vi "RichToFlatni_measurementlink_pinmap_v1_PinGroupDefinition.vi"(5 "OutputClusterType":T1, 11 "InputCluster":T2) -> (3 "OutputCluster":T1)   [LabVIEW 2021, in "ni.measurementlink.pinmap.v1.api.lvlib"]
uses:
  ni.measurementlink.pinmap.v1.api.lvlib
  ni_measurementlink_pinmap_v1_PinGroupDefinition.ctl
  ni_measurementlink_pinmap_v1_PinGroupDefinition_Flat.ctl
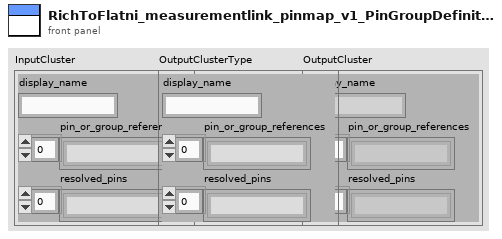
[diagram p1: front panel]
types:
  T1 = typedef "ni.measurementlink.pinmap.v1.api.lvlib/ni_measurementlink_pinmap_v1_PinGroupDefinition_Flat.ctl" = cluster{"display_name":string, "pin_or_group_references":string[], "resolved_pins":string[]}
  T2 = typedef "ni.measurementlink.pinmap.v1.api.lvlib/ni_measurementlink_pinmap_v1_PinGroupDefinition.ctl" = cluster{"display_name":string, "pin_or_group_references":string[], "resolved_pins":string[]}
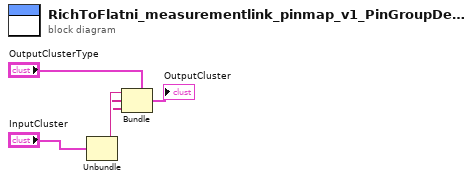
[diagram p0: block diagram]
diagram:
  n1 = Unbundle "Unbundle"("InputCluster") -> ("display_name"=w3:string, "pin_or_group_references"=w2:string[], "resolved_pins"=w1:string[])
  n2 = Bundle "Bundle"(cluster="OutputClusterType", "display_name"=w3, "pin_or_group_references"=w2, "resolved_pins"=w1) -> (→"OutputCluster":T1)
